vi "WriteFile.vi"(8 "error in (no error)":errorcluster, 10 "data":i32[](array[numeric]), 11 "WriteOnly in":refnum<class "WriteOnly.lvclass">) -> (0 "error out":errorcluster, 3 "WriteOnly out":refnum<class "WriteOnly.lvclass">)   [LabVIEW 2021]
uses:
  Interfaces/WriteOnly/WriteOnly.lvclass
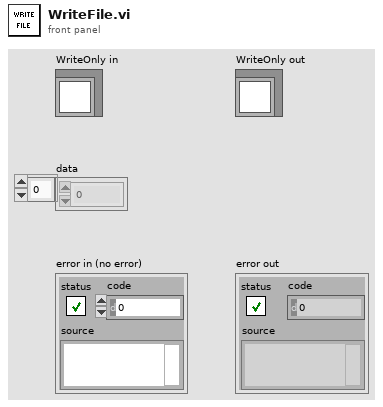
[diagram p1: front panel]
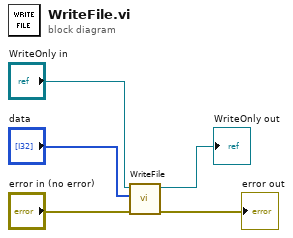
[diagram p0: block diagram]
diagram:
  n1 = call-dynamic "WriteFile.vi"("error in (no error)"="error in (no error)", "data"="data", "WriteOnly in"="WriteOnly in") -> ("error out"=→"error out":errorcluster, "WriteOnly out"=→"WriteOnly out":refnum<class "WriteOnly.lvclass">)  [unwired: 7 in]
